vi "内部交互全局.vi"() -> ()   [LabVIEW 2016, in "环境动力监测库.lvlib" / "智能门禁监测.lvlib"]
panel:
  out "门禁输出字符串":string
  out "门禁":bool
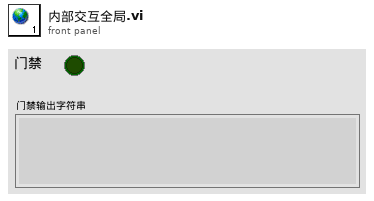
[diagram p1: front panel]
diagram:
